vi "Read Power.vi"(8 "error in":errorcluster, 11 "2936r in":refnum<class "2936r.lvclass">) -> (0 "error out":errorcluster, 3 "2936r out":refnum<class "2936r.lvclass">)   [LabVIEW 2017, in "2936r.lvlib" / "2936r.lvclass"]
uses:
  2936r.lvclass
  2936r.lvclass/2936r.ctl
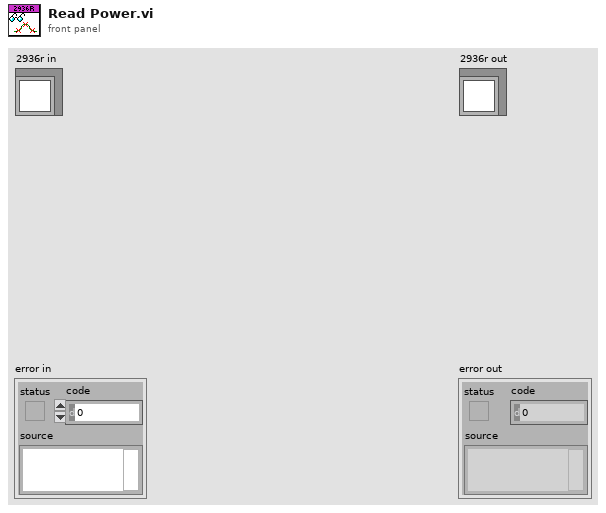
[diagram p1: front panel]
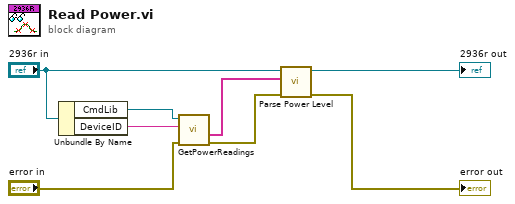
[diagram p0: block diagram]
diagram:
  n1 = Unbundle By Name("2936r in") -> ("CmdLib"=w8:refnum<k24>, "DeviceID"=w7:string)
  n2 = call <instrlib>:"GetPowerReadings.vi"("error in"="error in", "Device Key In"=w7, "PM Cmds In"=w8) -> ("error out"=w3:errorcluster, "Power Readings"=w4:string[])  [unwired: 1 in, 2 out]
  n3 = call "Parse Power Level.vi"("error in"=w3, "Read Values"=w4, "2936r in"="2936r in") -> ("error out"=→"error out":errorcluster, "2936r out"=→"2936r out":refnum<class "2936r.lvclass">)  [unwired: 7 in]
